vi "Main.vi"() -> ()   [LabVIEW 2020]
uses:
  Serial Settings.ctl
  Data Cluster.ctl
  Main Events.ctl
  <vilib>/Utility/NIReport.llb/Report Type.ctl
  bd07f4a1-b671-4ede-a250-6e16bfbd43fa.vi
  <vilib>/Instr/_visa.llb/VISA Configure Serial Port (Instr).vi
  <vilib>/Utility/file.llb/Write Delimited Spreadsheet (string).vi
  <vilib>/addons/_office/excel.llb/Excel Get Data ([str]).vi
  <vilib>/Comparison/Equal/Equal Functor/Equal Functor.lvclass
  <vilib>/Utility/NIReport.llb/NI_report.lvclass
  <vilib>/Utility/NIReport.llb/NI_ReportGenerationCore.lvlib
  <vilib>/addons/_office/NI_ReportGenerationToolkit.lvlib
  <vilib>/Utility/NIReport.llb/Excel/NI_Excel.lvclass
panel:
  in  "Add Button":bool caption="Start Button"
  in  "Command Data":string
  in  "Select Command":string(combo)
  in  "Create Chain":bool
  in  "Import Script":path
  in  "Save Script Button":bool caption="Start Button"
  out "Imported Commands":string[][](array[string])
  out "CMD Array":T1[](array[typedef])
  out "Data file path":path
  out "Data":string[][](table)=[["Loop", "Step", "Command", "Opcode Sent", "Data Received", "Data Decoded", "Retries", "Time (ms)", "Error"]]
  in  "Timeout (ms)":dbl=1000.0
  out "Script":string[][](table)
  in  "Serial Settings":T2={"baud rate"=115200, "data bits"=8, "parity"=enum."None", "stop bits"=10, "flow control"=0} {"flow control" items=["None"=0, "XON/XOFF"=1, "RTS/CTS"=2, "DTR/DSR"=4]; "stop bits" items=["1.0"=10, "1.5"=15, "2.0"=20]; "data bits" min=5 max=8 step=1; "baud rate" items=["75"=75, "110"=110, "134"=134, "150"=150, "300"=300, "600"=600, "1200"=1200, "1800"=1800, "2400"=2400, "4800"=4800, "7200"=7200, "9600"=9600, "14400"=14400, "19200"=19200, "28800"=28800, "38400"=38400, "56000"=56000, "57600"=57600, "115200"=115200, "128000"=128000, "230400"=230400]}
  in  "Stop Button":bool caption="Start Button"
  in  "Clear Button":bool caption="Start Button"
  out "Status":string
  in  "Start Button":bool
  in  "Number of Retries":u16=3
  in  "Number of Loops":u16=1
  out "COM Port LED":bool
  in  "Select COM Port":refnum<visa-resource-name>
  out "error out":errorcluster
  in  "error in":errorcluster
  # "Create Scipt"
  # "Send Data:"
  # "Receive Data:"
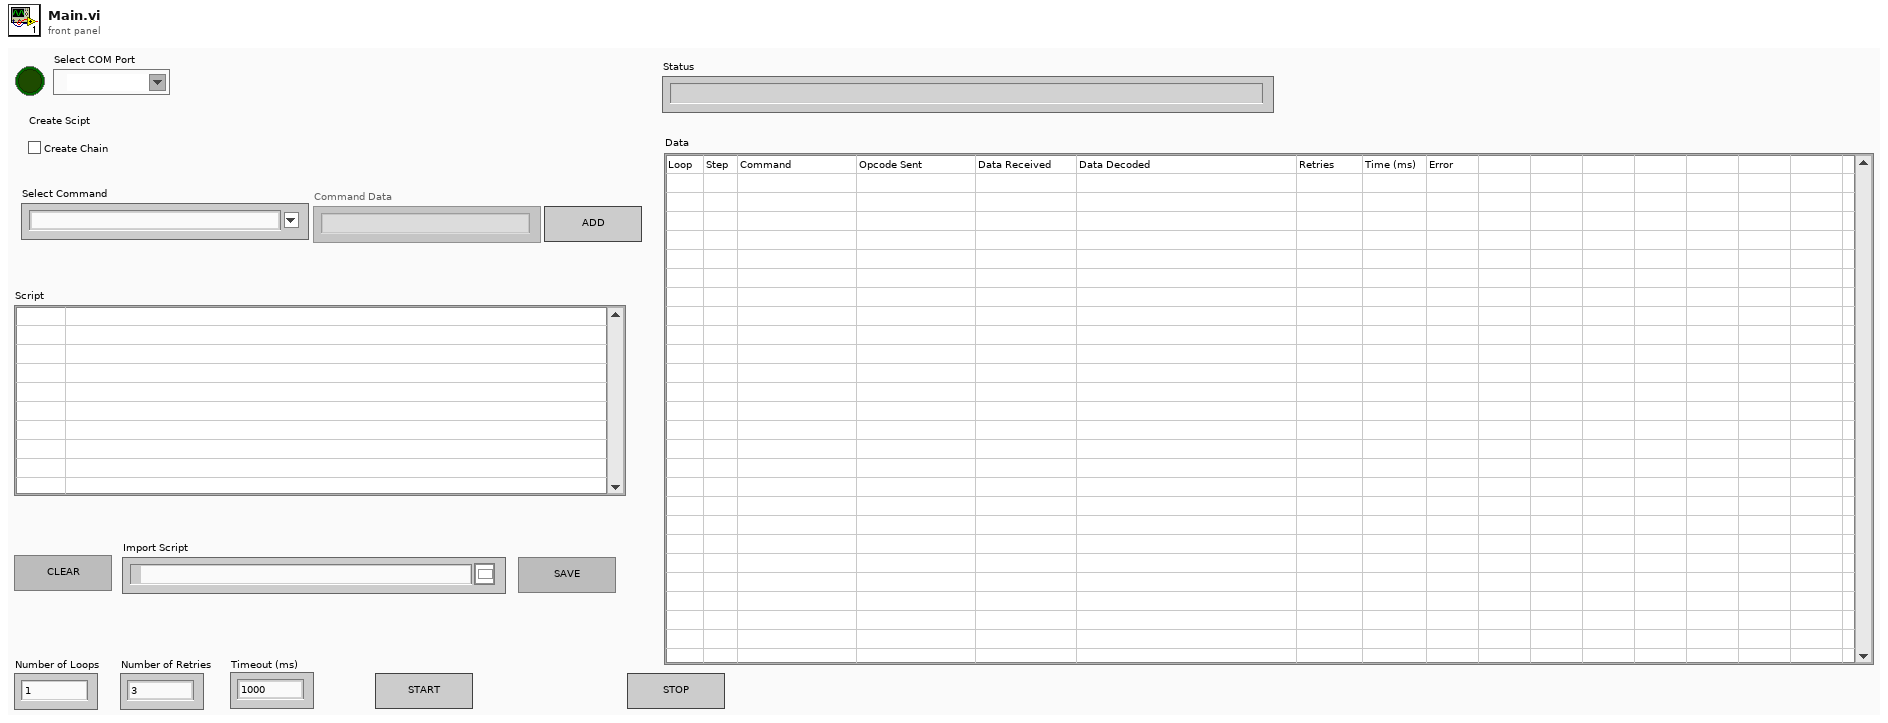
[diagram p1: front panel]
types:
  T1 = typedef "Data Cluster.ctl" = cluster{"Command Name":string, "Command Opcode ":string, "Step":dbl, "Loop":dbl, "Expected Response Size (bytes)":u16, "Number of cmds":dbl, "Data Received (byte array)":u8[], "Retries Executed":u16, "Time (ms)":u16, "Pass?":bool, "Opcode (off) / Instruction (on)":bool, "Data Received String (decoded)":string, "Error":string}
  T2 = typedef "Serial Settings.ctl" = cluster{"baud rate":u32, "data bits":u16, "parity":enum16{"None", "Odd", "Even", "Mark", "Space"}, "stop bits":u16, "flow control":u16}
  T3 = typedef "Main Events.ctl" = enum16{"Default", "Initialize cmds", "Initialize Data File", "Initialize COM Port", "Run Commands", "Save Data File", "End"}
  T4 = typedef "NI_ReportGenerationCore.lvlib/Report Type.ctl" = enum16{"HTML", "Word", "Excel"}
  T5 = enum8{"Enabled", "Disabled", "Disabled and Grayed Out"}
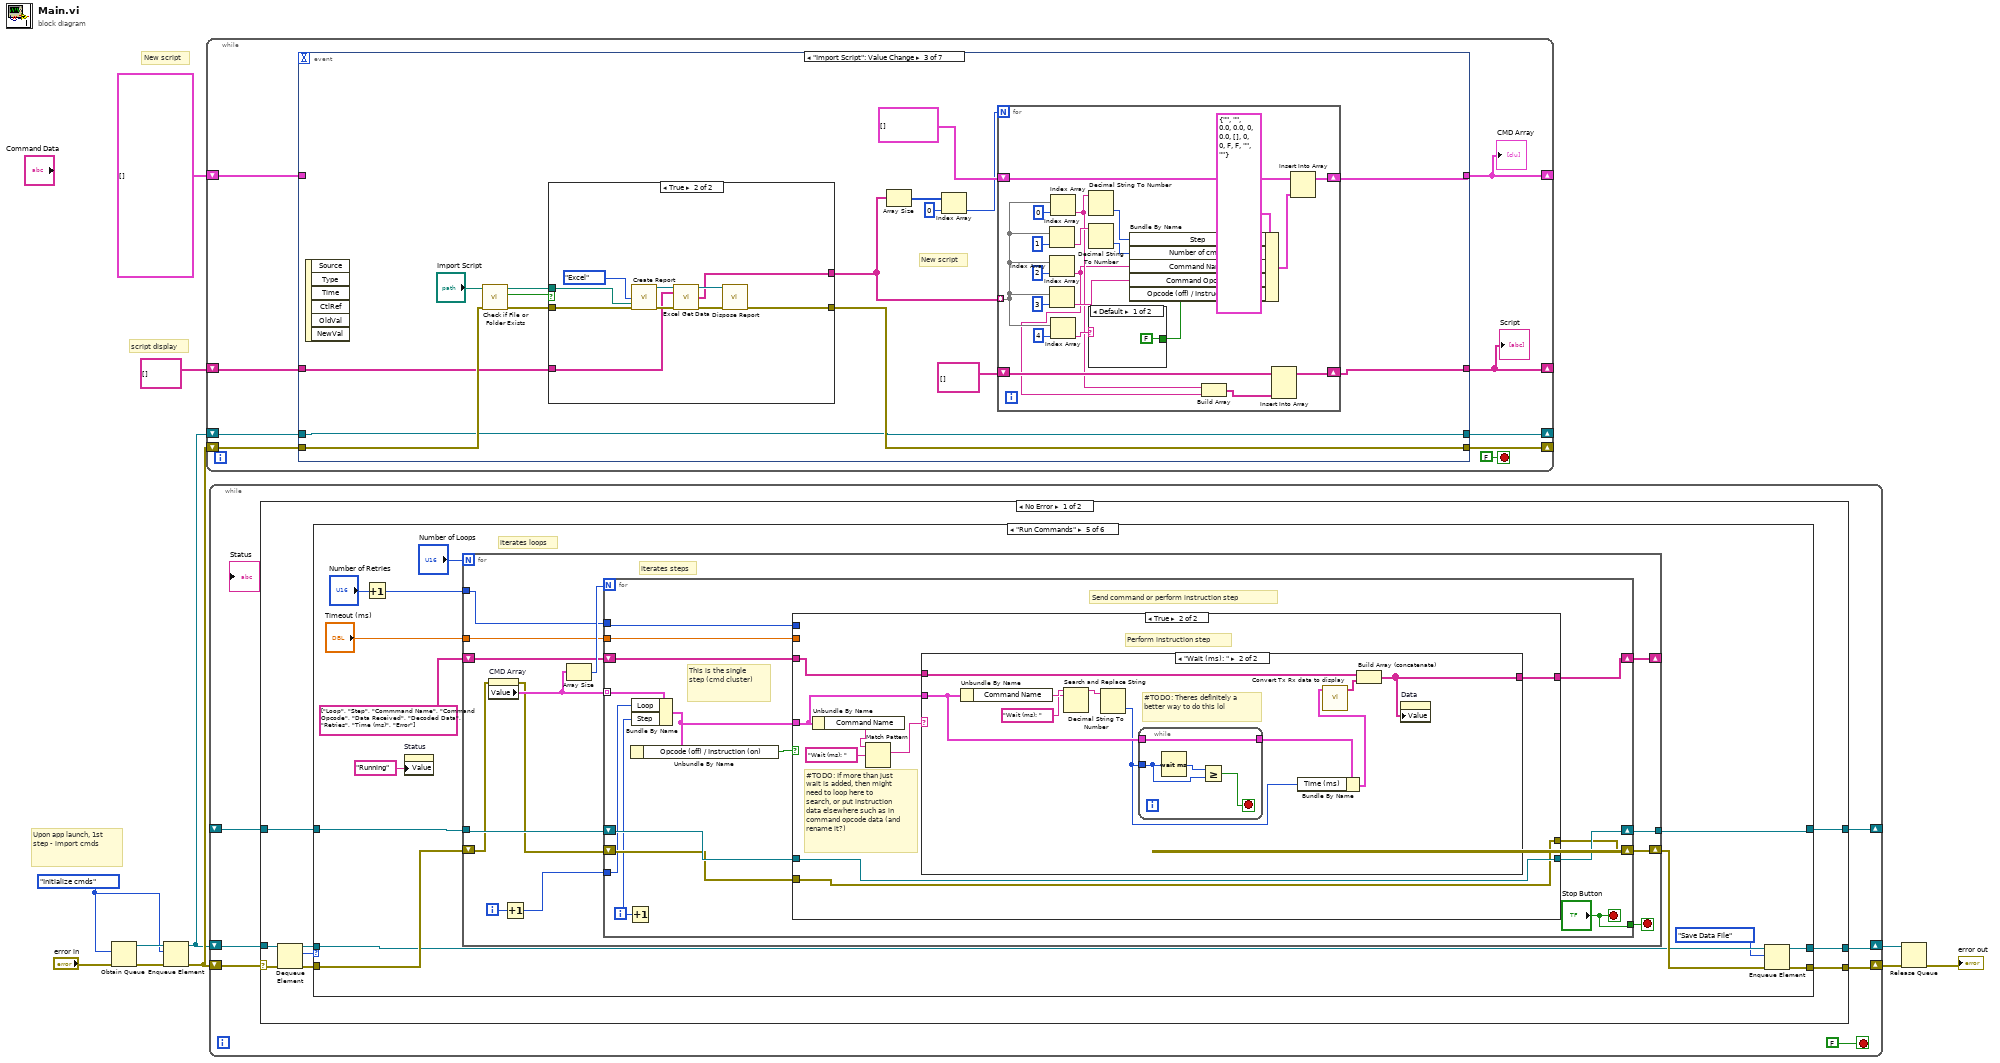
[diagram p0: block diagram]
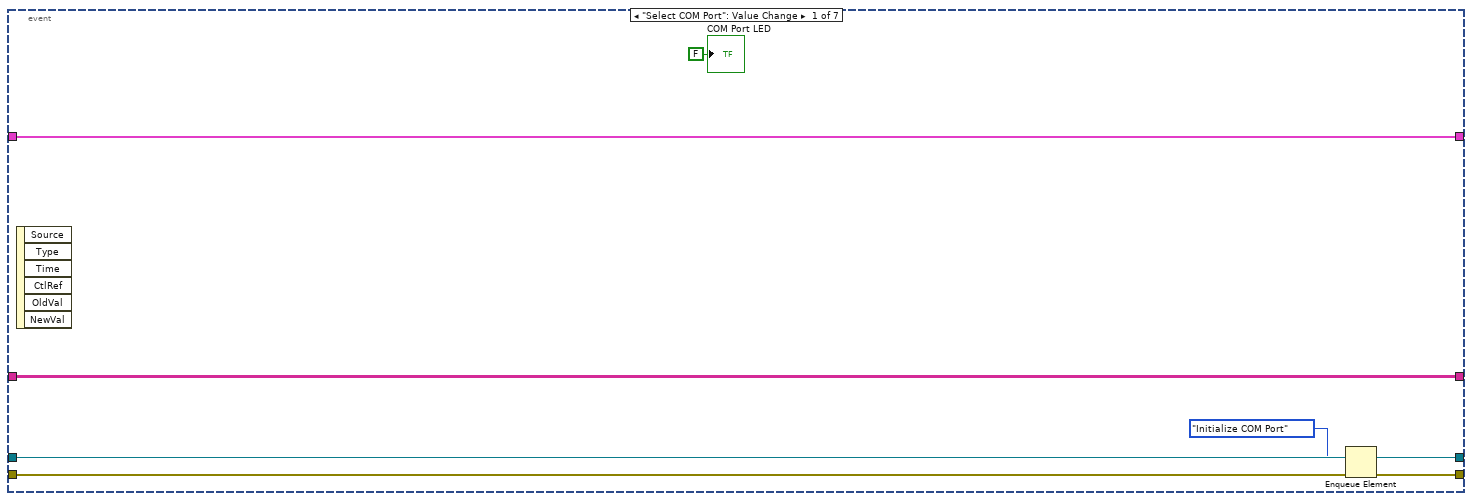
[diagram p2: hidden frame]
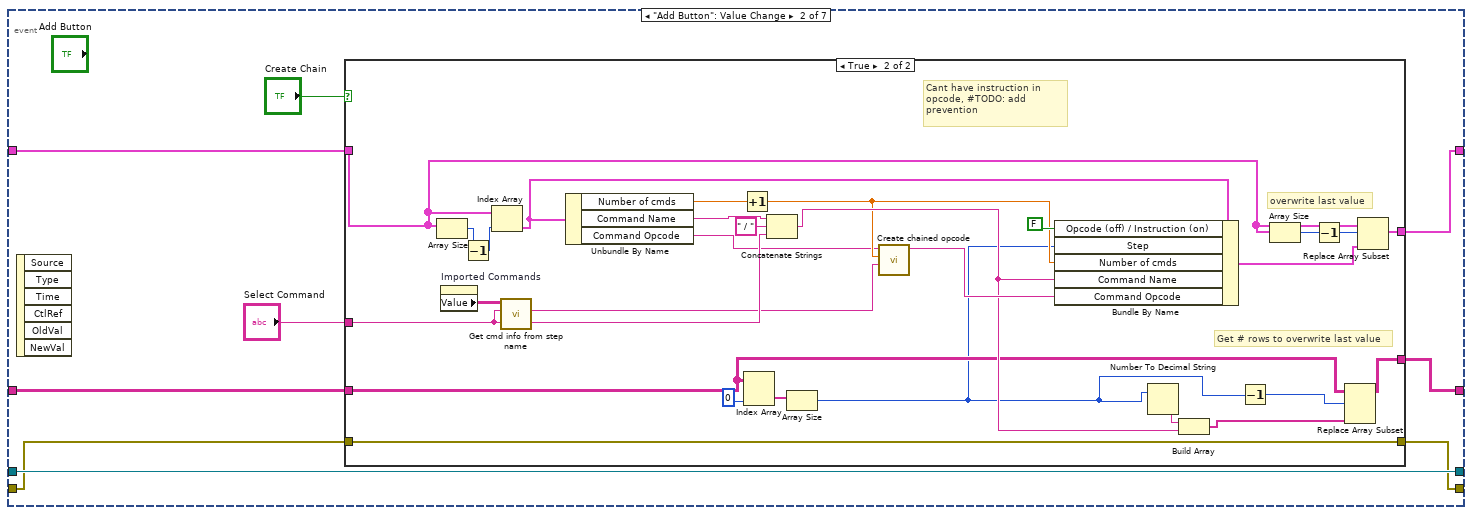
[diagram p3: hidden frame]
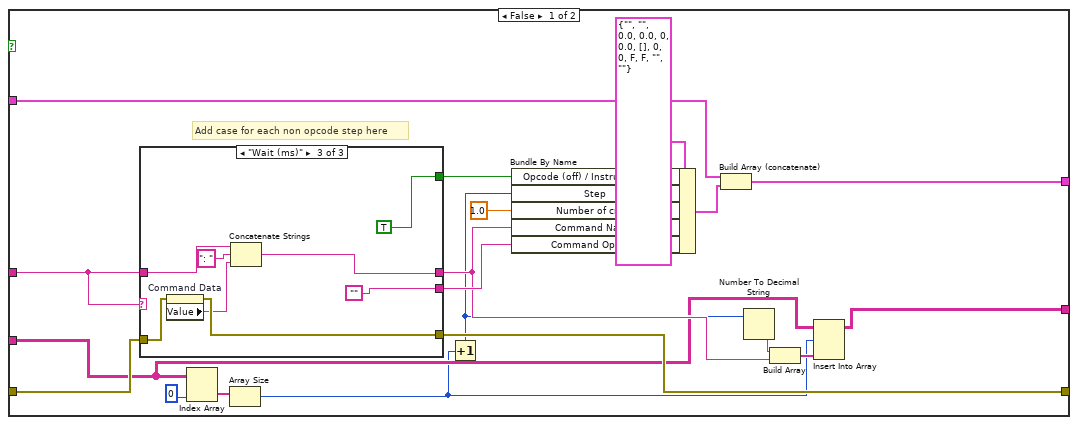
[diagram p4: hidden frame]
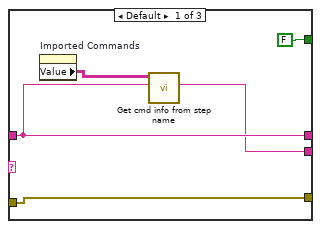
[diagram p5: hidden frame]
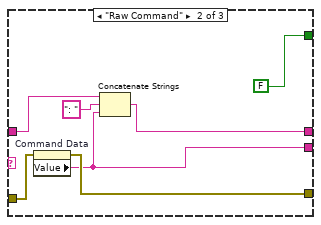
[diagram p6: hidden frame]
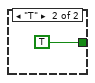
[diagram p7: hidden frame]
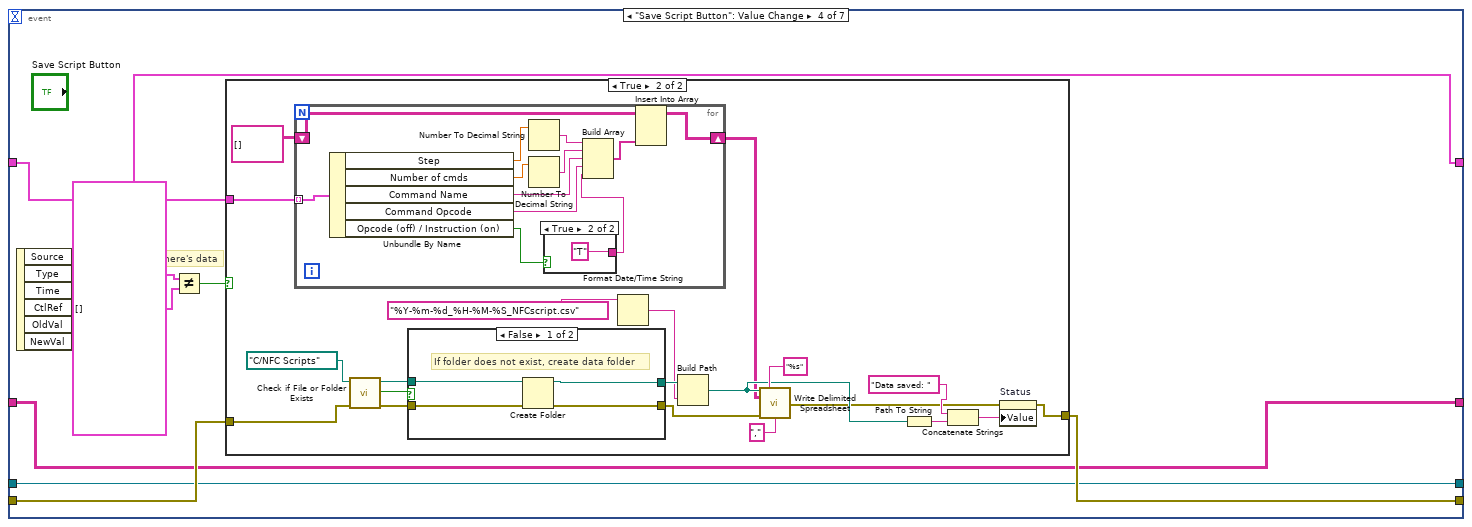
[diagram p9: hidden frame]
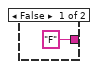
[diagram p11: hidden frame]
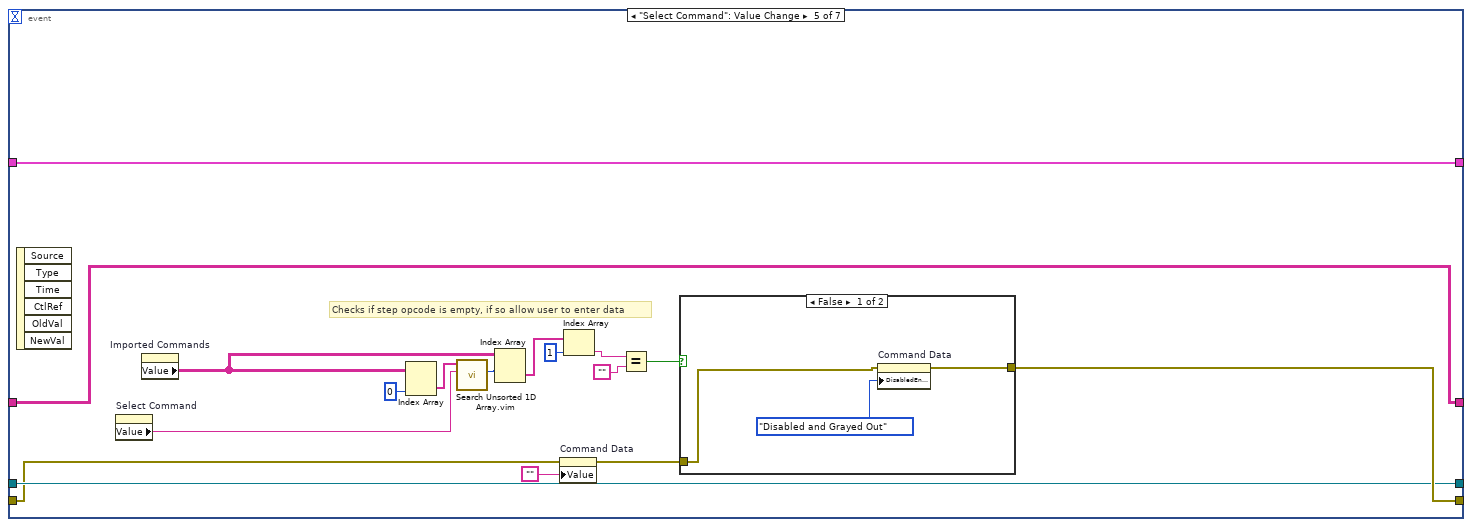
[diagram p13: hidden frame]
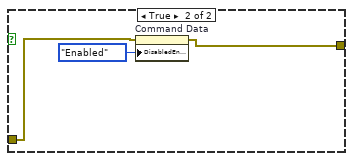
[diagram p14: hidden frame]
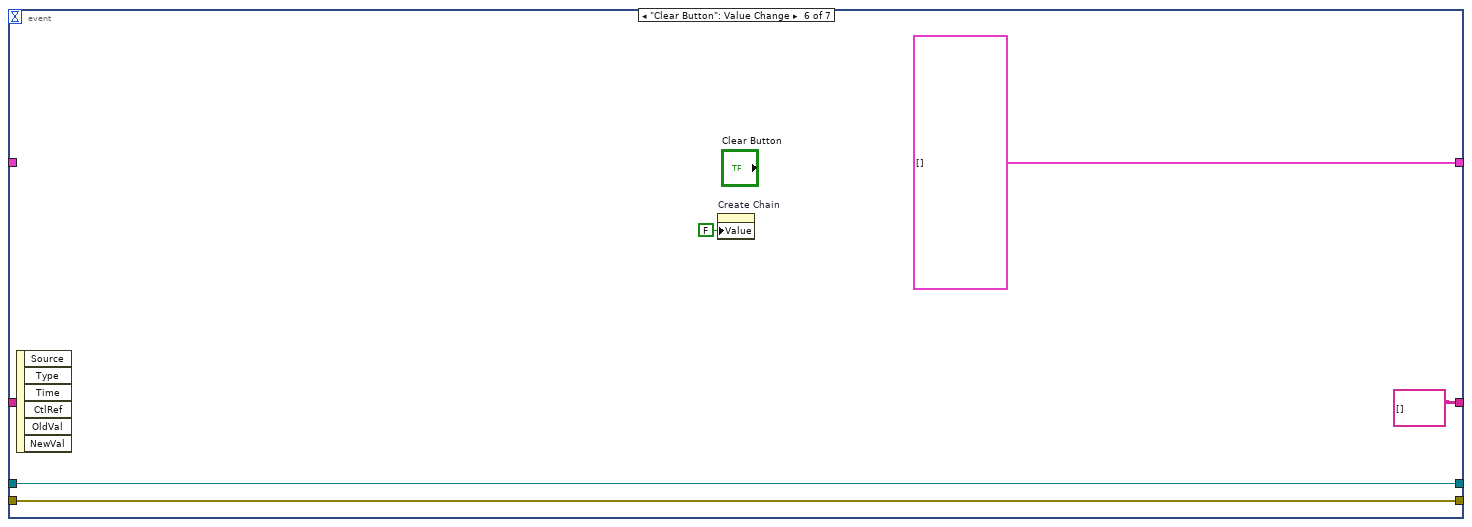
[diagram p15: hidden frame]
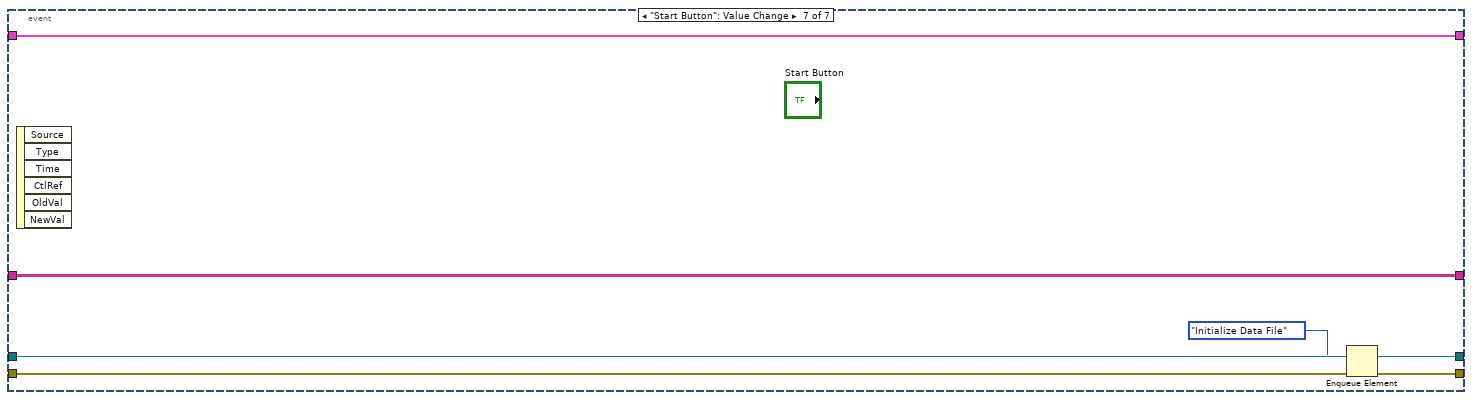
[diagram p16: hidden frame]
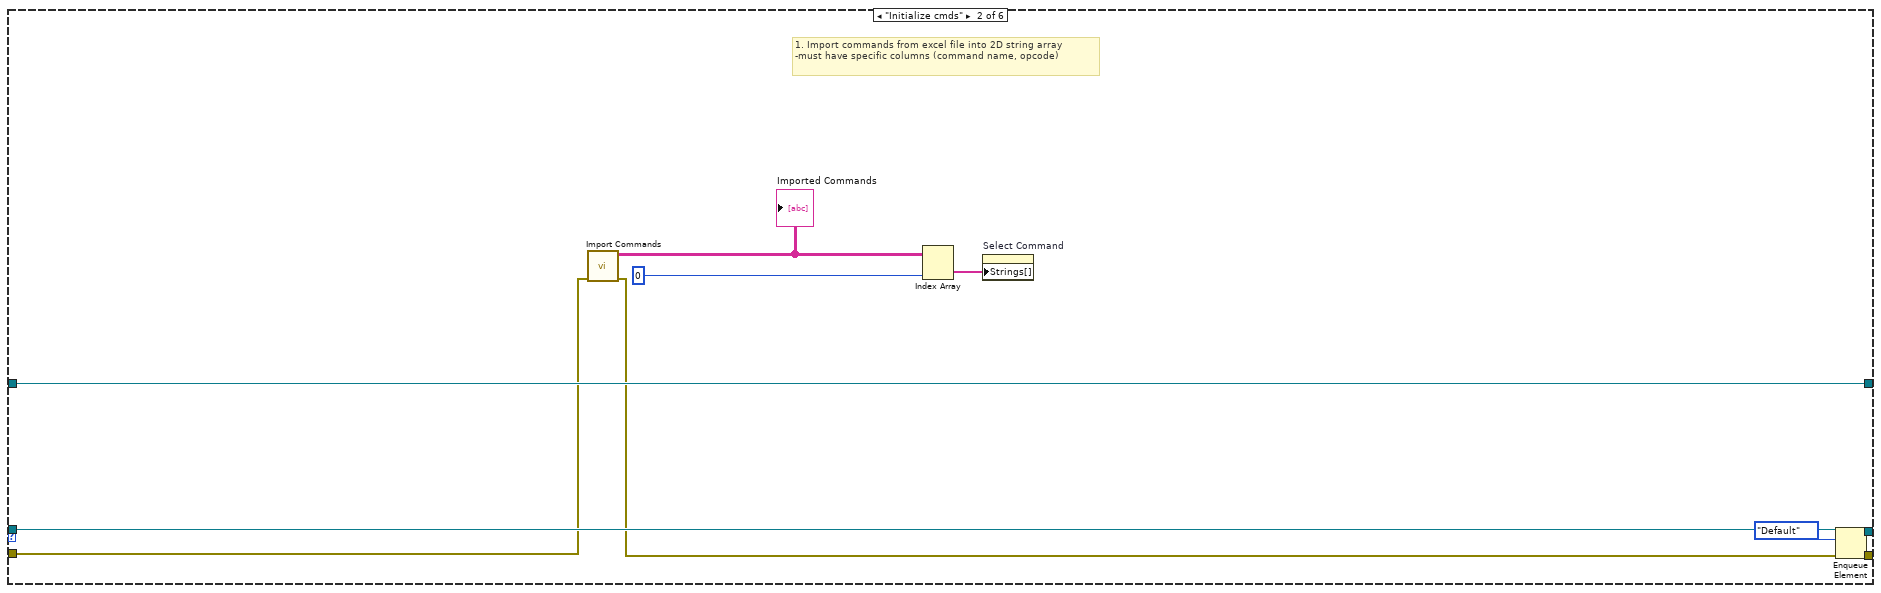
[diagram p18: hidden frame]
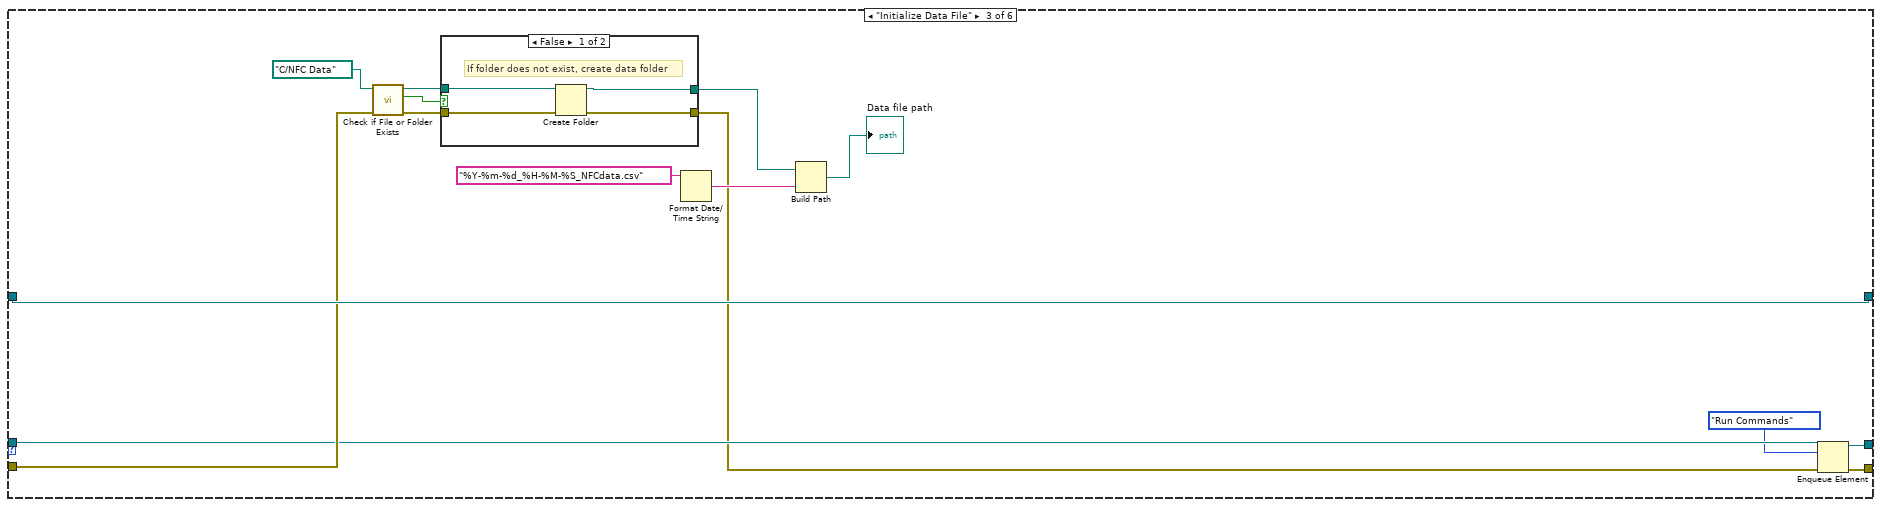
[diagram p19: hidden frame]
diagram:
  w3 = Main_Events."Initialize cmds" ("Main Enum")
  # "script display"
  # "New script"
  # "Upon app launch, 1st step - import cmds"
  n1 = Obtain Queue(element data type=w3, error in (no error)="error in") -> (queue out=w7:refnum<queue>, error out=w10:errorcluster)  [unwired: 3 in, 1 out]
  n2 = Enqueue Element(queue=w7, element=w3, error in (no error)=w10) -> (queue out=w4:refnum<queue>, error out=w5:errorcluster)  [unwired: 1 in, 1 out]
  n3 = while {
    shift-right: [w19] -> _
    shift-left: w5 -> [w20]
    shift-right: [w17] -> _
    shift-left: w4 -> [w18]
    shift-right: [w12] -> _
    shift-left: T1[] [] ("Array") -> [w15]
    shift-right: [w13] -> _
    shift-left: string[][] [] ("Script") -> [w14]
    stop <- FALSE stop-if-true
    n4 = event shown="[2] \"Import Script\": Value Change" {
      selector: _ -> [_ _ _ _ _ _ _]
      dyn-events: _ -> [_ _ _ _ _ _ _]
      timeout: _ -> [_ _ _ _ _ _ _]
      tunnel: w20 -> [w24 w34 w116 w161 w205 w229 w236]
      tunnel: [w28 w33 w114 w160 w220 w229 w237] -> w19
      tunnel: w18 -> [w27 w35 w113 w159 w219 w230 w235]
      tunnel: [w26 w35 w113 w159 w219 w230 w238] -> w17
      tunnel: w15 -> [w22 w32 _ w156 w218 _ w233]
      tunnel: [w22 w31 w110 w156 w218 T1[] [] ("Array") w233] -> w12
      tunnel: w14 -> [w21 w30 w115 w158 w217 _ w232]
      tunnel: [w21 w29 w108 w158 w217 string[][] [] ("Script") w232] -> w13
      event "Select COM Port": Value Change {
        n5 = event-data() -> ()  [unwired: 1 in, 6 out]
        n6 = Enqueue Element(queue=w27, element=Main_Events."Initialize COM Port" ("Main Enum"), error in (no error)=w24) -> (queue out=w26:refnum<queue>, error out=w28:errorcluster)  [unwired: 1 in, 1 out]
        "COM Port LED" <- FALSE ("COM Port LED")
      }
      event "Add Button": Value Change {
        n7 = event-data() -> ()  [unwired: 1 in, 6 out]
        n8 = case shown="True" "Create Chain" {
          tunnel: "Select Command" -> [w56 w83]
          tunnel: w34 -> [w55 w103]
          tunnel: [w54 w103] -> w33
          tunnel: w32 -> [w48 w99]
          tunnel: [w47 w97] -> w31
          tunnel: w30 -> [w40 w88]
          tunnel: [w39 w89] -> w29
          frame False {
            # "Add case for each non opcode step here"
            n9 = case shown="\"Wait (ms)\"" w56 {
              tunnel: [w58 w66 w74] -> w44
              tunnel: w56 -> [w58 w68 w76]
              tunnel: [w57 w63 ""] -> w51
              tunnel: w55 -> [w61 w65 w73]
              tunnel: [w61 w64 w72] -> w54
              tunnel: [FALSE ("Opcode (off) / Instruction (on)") FALSE ("Opcode (off) / Instruction (on)") TRUE ("Opcode (off) / Instruction (on)")] -> w50
              frame Default {
                n10 = property on="Imported Commands" class="Arr (strict)"() -> ("Value"=w59:string[][])  [unwired: 2 in, 2 out]
                n11 = call "Get cmd info from step name.vi"("Select Command"=w58, "Command Library Data"=w59) -> ("cmd opcode (string)"=w57:string)  [unwired: 8 in, 1 out]
              }
              frame "Raw Command" {
                n12 = property on="Command Data" class="Str"(error in=w65) -> (error out=w64:errorcluster, "Value"=w63:string)  [unwired: 1 in, 1 out]
                n13 = Concatenate Strings(w68, ": " ("string"), w63) -> (w66:string)
              }
              frame "Wait (ms)" {
                n14 = property on="Command Data" class="Str"(error in=w73) -> (error out=w72:errorcluster, "Value"=w71:string)  [unwired: 1 in, 1 out]
                n15 = Concatenate Strings(w76, ": " ("string"), w71) -> (w74:string)
              }
            }
            n16 = Index Array(array=w40, index (col)=0 ("index")) -> (element=w42:string[])  [unwired: 1 in]
            n17 = Array Size(array=w42) -> (size(s)=w38:i32)
            n18 = Increment(x=w38) -> (x+1=w41:i32)
            n19 = Bundle By Name(cluster=T1 {"Command Name"="", "Command Opcode "="", "Step"=0.0, "Loop"=0.0, "Expected Response Size (bytes)"=0, "Number of cmds"=0.0, "Data Received (byte array)"=[], "Retries Executed"=0, "Time (ms)"=0, "Pass?"=FALSE, "Opcode (off) / Instruction (on)"=FALSE, "Data Received String (decoded)"="", "Error"=""} ("Data Cluster"), "Opcode (off) / Instruction (on)"=w50, "Step"=w41, "Number of cmds"=1.0, "Command Name"=w44, "Command Opcode"=w51) -> (w53:T1)
            n20 = Build Array (concatenate)(w48, w53) -> (w47:T1[])
            n21 = Number To Decimal String(number=w41) -> (decimal integer string=w46:string)  [unwired: 1 in]
            n22 = Build Array(w46, w44) -> (w45:string[])
            n23 = Insert Into Array(array=w40, index (row)=w38, new element=w45) -> (w39:string[][])  [unwired: 1 in]
          }
          frame True {
            # "Cant have instruction in opcode, #TODO: add prevention"
            # "Get # rows to overwrite last value"
            # "overwrite last value"
            n24 = Array Size(array=w99) -> (size(s)=w93:i32)
            n25 = property on="Imported Commands" class="Arr (strict)"() -> ("Value"=w84:string[][])  [unwired: 2 in, 2 out]
            n26 = Decrement(x=w93) -> (x-1=w92:i32)
            n27 = Index Array(array=w99, index=w92) -> (element=w96:T1)
            n28 = call "Get cmd info from step name.vi"("Select Command"=w83, "Command Library Data"=w84) -> ("cmd opcode (string)"=w81:string)  [unwired: 8 in, 1 out]
            n29 = Unbundle By Name(w96) -> ("Number of cmds"=w82:dbl, "Command Name"=w102:string, "Command Opcode"=w79:string)
            n30 = Increment(x=w82) -> (x+1=w80:dbl)
            n31 = Index Array(array=w88, index (col)=0 ("index")) -> (element=w86:string[])  [unwired: 1 in]
            n32 = Concatenate Strings(w102, " / " ("string"), w83) -> (w90:string)
            n33 = Array Size(array=w86) -> (size(s)=w78:i32)
            n34 = call "Create chained opcode.vi"("new cmd opcode"=w81, "Number of commands"=w80, "Current cmd opcode"=w79) -> ("new chained opcode"=w100:string)  [unwired: 8 in]
            n35 = Bundle By Name(cluster=w96, "Opcode (off) / Instruction (on)"=FALSE, "Step"=w78, "Number of cmds"=w80, "Command Name"=w90, "Command Opcode"=w100) -> (w98:T1)
            n36 = Number To Decimal String(number=w78) -> (decimal integer string=w91:string)  [unwired: 1 in]
            n37 = Build Array(w91, w90) -> (w85:string[])
            n38 = Decrement(x=w78) -> (x-1=w77:i32)
            n39 = Array Size(array=w99) -> (size(s)=w95:i32)
            n40 = Decrement(x=w95) -> (x-1=w94:i32)
            n41 = Replace Array Subset(array=w88, new element=w85, index (row)=w77) -> (w89:string[][])  [unwired: 1 in]
            n42 = Replace Array Subset(array=w99, new element=w98, index=w94) -> (w97:T1[])
          }
        }
      }
      event "Import Script": Value Change {
        # "New script"
        n43 = event-data() -> ()  [unwired: 1 in, 6 out]
        n44 = call <vilib>:"Check if File or Folder Exists.vi"("error in (no error)"=w116, "path"="Import Script") -> ("error out"=w117:errorcluster, "file or folder exists?"=w119:bool, "dup path"=w118:path)  [unwired: 7 in]
        n45 = case shown="True" w119 {
          tunnel: [w144 w146] -> w107
          tunnel: [w145 w154] -> w114
          tunnel: w118 -> [_ w149]
          tunnel: w117 -> [w145 w148]
          tunnel: w115 -> [w144 w147]
          frame False {
          }
          frame True {
            n46 = call <vilib>:"Create Report.vi"("report type"=Report_Type."Excel", "template (empty)"=w149, "error in (no error)"=w148) -> ("report out"=w153:refnum<class "NI_report.lvclass">, "error out"=w151:errorcluster)  [unwired: 11 in]
            n47 = call-poly <vilib>:"Excel Get Data.vi"("report in"=w153, "data type"=w147, "error in (no error)"=w151) -> ("report out"=w152:refnum<class "NI_report.lvclass">, "data"=w146:string[][], "error out"=w150:errorcluster)  [unwired: 10 in]
            n48 = call-dynamic "Dispose Report.vi"("report in"=w152, "error in (no error)"=w150) -> ("error out"=w154:errorcluster)  [unwired: 13 in]
          }
        }
        n49 = Array Size(array=w107) -> (size(s)=w106:i32[])
        n50 = Index Array(array=w106, index=0) -> (element=w105:i32)
        n51 = for {
          N: w105 -> [_]
          tunnel: w107 -> [w136] mode=indexing
          shift-right: [w126] -> w110
          shift-left: T1[] [] ("Array") -> [w128]
          shift-right: [w125] -> w108
          shift-left: string[][] [] ("Script") -> [w124]
          n52 = Index Array(array=w136, index=1) -> (element=w133:string)
          n53 = Index Array(array=w136, index=2) -> (element=w122:string)
          n54 = Index Array(array=w136, index=3) -> (element=w134:string)
          n55 = Index Array(array=w136, index=0) -> (element=w123:string)
          n56 = Index Array(array=w136, index=4) -> (element=w130:string)
          n57 = Decimal String To Number(string=w123) -> (number=w131:i32)  [unwired: 2 in, 1 out]
          n58 = Decimal String To Number(string=w133) -> (number=w132:i32)  [unwired: 2 in, 1 out]
          n59 = case shown="Default" w130 {
            tunnel: [FALSE TRUE] -> w129
            frame Default {
            }
            frame "T" {
            }
          }
          n60 = Bundle By Name(cluster=T1 {"Command Name"="", "Command Opcode "="", "Step"=0.0, "Loop"=0.0, "Expected Response Size (bytes)"=0, "Number of cmds"=0.0, "Data Received (byte array)"=[], "Retries Executed"=0, "Time (ms)"=0, "Pass?"=FALSE, "Opcode (off) / Instruction (on)"=FALSE, "Data Received String (decoded)"="", "Error"=""} ("Data Cluster"), "Step"=w131, "Number of cmds"=w132, "Command Name"=w122, "Command Opcode"=w134, "Opcode (off) / Instruction (on)"=w129) -> (w127:T1)
          n61 = Build Array(w123, w122) -> (w121:string[])
          n62 = Insert Into Array(array=w124, new element=w121) -> (w125:string[][])  [unwired: 2 in]
          n63 = Insert Into Array(array=w128, new element=w127) -> (w126:T1[])  [unwired: 1 in]
        }
      }
      event "Save Script Button": Value Change {
        # "If there's data"
        n64 = event-data() -> ()  [unwired: 1 in, 6 out]
        n65 = Not Equal?(x=w156, y=T1[] [] ("Array")) -> (x != y?=w162:bool)
        n66 = case shown="True" w162 {
          tunnel: w161 -> [w163 w176]
          tunnel: [w163 w167] -> w160
          tunnel: w156 -> [_ w166]
          frame False {
          }
          frame True {
            n67 = for {
              tunnel: w166 -> [w195] mode=indexing
              shift-right: [w192] -> w164
              shift-left: string[][] [] ("Script") -> [w193]
              n68 = Unbundle By Name(w195) -> ("Step"=w191:dbl, "Number of cmds"=w190:dbl, "Command Name"=w187:string, "Command Opcode"=w186:string, "Opcode (off) / Instruction (on)"=w185:bool)
              n69 = Number To Decimal String(number=w191) -> (decimal integer string=w189:string)  [unwired: 1 in]
              n70 = Number To Decimal String(number=w190) -> (decimal integer string=w188:string)  [unwired: 1 in]
              n71 = case shown="True" w185 {
                tunnel: ["F" "T"] -> w184
                frame False {
                }
                frame True {
                }
              }
              n72 = Build Array(w189, w188, w187, w186, w184) -> (w194:string[])
              n73 = Insert Into Array(array=w193, new element=w194) -> (w192:string[][])  [unwired: 2 in]
            }
            n74 = call <vilib>:"Check if File or Folder Exists.vi"("error in (no error)"=w176, "path"=path "C:/NFC Scripts") -> ("error out"=w181:errorcluster, "file or folder exists?"=w183:bool, "dup path"=w182:path)  [unwired: 7 in]
            n75 = case shown="False" w183 {
              tunnel: w182 -> [w201 w203]
              tunnel: w181 -> [w200 w202]
              tunnel: [w199 w203] -> w179
              tunnel: [w198 w202] -> w171
              frame False {
                # "If folder does not exist, create data folder"
                n76 = Create Folder(path (use dialog)=w201, error in=w200) -> (created path=w199:path, error out=w198:errorcluster)  [unwired: 1 in, 1 out]
              }
              frame True {
              }
            }
            n77 = Format Date/Time String(time format string (%c)="%Y-%m-%d_%H-%M-%S_NFCscript.csv") -> (date/time string=w178:string)  [unwired: 2 in]
            n78 = Build Path(base path=w179, name or relative path=w178) -> (appended path=w170:path)
            n79 = call-poly <vilib>:"Write Delimited Spreadsheet.vi"("file path (dialog if empty)"=w170, "format (%s)"="%s", "2D data"=w164, "error in (no error)"=w171, "delimiter (\\t)"="," ("delimiter (\\t)")) -> ("error out"=w169:errorcluster)  [unwired: 9 in, 1 out]
            n80 = Path To String(path=w170) -> (string=w173:string)
            n81 = Concatenate Strings("Data saved: " ("Status"), w173) -> (w168:string)
            n82 = property on="Status" class="Str"(error in=w169, "Value"=w168) -> (error out=w167:errorcluster)  [unwired: 1 in, 1 out]
          }
        }
      }
      event "Select Command": Value Change {
        # "Checks if step opcode is empty, if so allow user to enter data"
        n83 = event-data() -> ()  [unwired: 1 in, 6 out]
        n84 = property on="Select Command" class="CmbBox"() -> ("Value"=w210:string)  [unwired: 2 in, 2 out]
        n85 = property on="Imported Commands" class="Arr (strict)"() -> ("Value"=w211:string[][])  [unwired: 2 in, 2 out]
        n86 = Index Array(array=w211, index (col)=0 ("disabled index (col)")) -> (element=w215:string[])  [unwired: 1 in]
        n87 = call "Search Unsorted 1D Array.vim"("element"=w210, "unsorted 1D array"=w215) -> ("index of element"=w216:i32)  [unwired: 9 in]
        n88 = Index Array(array=w211, index (row)=w216) -> (element=w212:string[])  [unwired: 1 in]
        n89 = property on="Command Data" class="Str"(error in=w205, "Value"="") -> (error out=w204:errorcluster)  [unwired: 1 in, 1 out]
        n90 = Index Array(array=w212, index=1) -> (element=w209:string)
        n91 = Equal?(x=w209, y="") -> (x = y?=w207:bool)
        n92 = case shown="False" w207 {
          tunnel: w204 -> [w221 w225]
          tunnel: [w222 w224] -> w220
          frame False {
            n93 = property on="Command Data" class="Str"(error in=w221, "DisabledEnum"=T5."Disabled and Grayed Out" ("Disabled")) -> (error out=w222:errorcluster)  [unwired: 1 in, 1 out]
          }
          frame True {
            n94 = property on="Command Data" class="Str"(error in=w225, "DisabledEnum"=T5."Enabled" ("Disabled")) -> (error out=w224:errorcluster)  [unwired: 1 in, 1 out]
          }
        }
      }
      event "Clear Button": Value Change {
        n95 = event-data() -> ()  [unwired: 1 in, 6 out]
        n96 = property on="Create Chain" class="Bool (strict)"("Value"=FALSE ("Create Chain")) -> ()  [unwired: 2 in, 2 out]
      }
      event "Start Button": Value Change {
        n97 = event-data() -> ()  [unwired: 1 in, 6 out]
        n98 = Enqueue Element(queue=w235, element=Main_Events."Initialize Data File", error in (no error)=w236) -> (queue out=w238:refnum<queue>, error out=w237:errorcluster)  [unwired: 1 in, 1 out]
      }
    }
    "Script" <- w13
    "CMD Array" <- w12
  }
  n99 = while {
    shift-right: [w243] -> w9
    shift-left: w5 -> [w245]
    shift-right: [w242] -> w6
    shift-left: w4 -> [w244]
    shift-right: [w241] -> _
    shift-left: _ -> [w240]
    stop <- FALSE stop-if-true
    n100 = case shown="No Error" w245 {
      selector: w245 -> [w253 w427]
      tunnel: w244 -> [w252 w428]
      tunnel: [w249 w427] -> w243
      tunnel: [w248 w428] -> w242
      tunnel: [w247 w426] -> w241
      tunnel: w240 -> [w246 w426]
      frame No Error {
        n101 = Dequeue Element(queue=w252, error in (no error)=w253) -> (queue out=w250:refnum<queue>, element=w251:T3, error out=w254:errorcluster)  [unwired: 1 in, 1 out]
        n102 = case shown="\"Run Commands\"" w251 {
          tunnel: w254 -> [w256 w262 w279 w300 w329 w422]
          tunnel: w250 -> [w257 w266 w272 w299 w324 w423]
          tunnel: [w256 w267 w273 w289 w326 w414] -> w249
          tunnel: [w257 w265 w274 w292 w327 w423] -> w248
          tunnel: [w255 w263 w282 w291 w330 w424] -> w247
          tunnel: w246 -> [w255 w263 w282 _ w331 w424]
          frame "Default", Default {
          }
          frame "Initialize cmds" {
            # "1. Import commands from excel file into 2D string array\n-must have specific columns (command name, opcode)"
            n103 = call "Import Commands.vi"("error in"=w262) -> ("error out"=w261:errorcluster, "Imported Commands"=w258:string[][])  [unwired: 9 in]
            "Imported Commands" <- w258
            n104 = Index Array(array=w258, index (col)=0 ("disabled index (col)")) -> (element=w259:string[])  [unwired: 1 in]
            n105 = property on="Select Command" class="CmbBox"("Strings[]"=w259) -> ()  [unwired: 2 in, 2 out]
            n106 = Enqueue Element(queue=w266, element=Main_Events."Default" ("Main Enum"), error in (no error)=w261) -> (queue out=w265:refnum<queue>, error out=w267:errorcluster)  [unwired: 1 in, 1 out]
          }
          frame "Initialize Data File" {
            n107 = call <vilib>:"Check if File or Folder Exists.vi"("error in (no error)"=w279, "path"=path "C:/NFC Data") -> ("error out"=w278:errorcluster, "file or folder exists?"=w281:bool, "dup path"=w280:path)  [unwired: 7 in]
            n108 = case shown="False" w281 {
              tunnel: w280 -> [w286 w288]
              tunnel: w278 -> [w285 w287]
              tunnel: [w284 w288] -> w276
              tunnel: [w283 w287] -> w268
              frame False {
                # "If folder does not exist, create data folder"
                n109 = Create Folder(path (use dialog)=w286, error in=w285) -> (created path=w284:path, error out=w283:errorcluster)  [unwired: 1 in, 1 out]
              }
              frame True {
              }
            }
            n110 = Format Date/Time String(time format string (%c)="%Y-%m-%d_%H-%M-%S_NFCdata.csv") -> (date/time string=w275:string)  [unwired: 2 in]
            n111 = Build Path(base path=w276, name or relative path=w275) -> (appended path=→"Data file path":path)
            n112 = Enqueue Element(queue=w272, element=Main_Events."Run Commands", error in (no error)=w268) -> (queue out=w274:refnum<queue>, error out=w273:errorcluster)  [unwired: 1 in, 1 out]
          }
          frame "Initialize COM Port" {
            # "If there's any error at this point, it's displayed and cleared. This assumes the error is com related and then clears all errors"
            # "Configure the serial port and wait 1 sec."
            n113 = Unbundle By Name("Serial Settings") -> ("baud rate"=w297:u32, "data bits"=w294:u16, "parity"=w296:enum16{"None", "Odd", "Even", "Mark", "Space"}, "stop bits"=w295:u16)
            n114 = call-poly "VISA Configure Serial Port"("VISA resource name"="Select COM Port", "Enable Termination\nChar (T)"=FALSE ("Enable Termination\nChar (T)"), "baud rate (9600)"=w297, "data bits (8)"=w294, "parity (0:none)"=w296, "error in (no error)"=w300, "stop bits (10: 1 bit)"=w295) -> ("VISA resource name out"=w298:refnum<visa-resource-name>, "error out"=w303:errorcluster)  [unwired: 7 in]
            n115 = call "Time Delay"("error in (no error)"=w303, "Delay Time (s)"=1.0) -> ("error out"=w290:errorcluster)  [unwired: 9 in]
            n116 = case shown="No Error" w290 {
              selector: w290 -> [w306 w311]
              tunnel: w299 -> [w309 w316]
              tunnel: [w305 w317] -> w289
              tunnel: [w309 w316] -> w292
              tunnel: [w308 refnum<visa-resource-name> refnum ("VISA resource name out")] -> w291
              tunnel: w298 -> [w308 w315]
              frame No Error {
                # "No COM Error... Continue"
                n117 = property on="COM Port LED" class="Bool (strict)"(error in=w306, "Value"=TRUE ("COM Port LED")) -> (error out=w305:errorcluster)  [unwired: 1 in, 1 out]
              }
              frame Error {
                n118 = property on="COM Port LED" class="Bool (strict)"(error in=w311, "Value"=FALSE ("COM Port LED")) -> (error out=w310:errorcluster)  [unwired: 1 in, 1 out]
                n119 = VISA Close(VISA resource name=w315, error in (no error)=w310) -> (error out=w314:errorcluster)
                n120 = call <vilib>:"Simple Error Handler.vi"("error in (no error)"=w314) -> ("error out"=w318:errorcluster)  [unwired: 4 in, 4 out]
                n121 = call <vilib>:"Clear Errors.vi"("error in (no error)"=w318) -> ("error out"=w317:errorcluster)  [unwired: 5 in, 1 out]
              }
            }
          }
          frame "Run Commands" {
            # "iterates loops"
            n122 = Increment(x="Number of Retries") -> (x+1=w320:u16)
            n123 = property on="Status" class="Str"("Value"="Running" ("Status")) -> ()  [unwired: 2 in, 2 out]
            n124 = for {
              N: "Number of Loops" -> [_]
              tunnel: [w345] -> w330
              tunnel: w331 -> [w343]
              shift-right: [w344] -> w325
              shift-left: w329 -> [w336]
              shift-right: [w339] -> _
              shift-left: string[][] [["Loop", "Step", "Commmand Name", "Command Opcode", "Data Received", "Decoded Data", "Retries", "Time (ms)", "Error"]] ("element") -> [w340]
              tunnel: w320 -> [w334]
              tunnel: "Timeout (ms)" -> [w333]
              i -> [w342]
              stop <- w338 stop-if-true
              # "iterates steps"
              n125 = property on="CMD Array" class="Arr (strict)"(error in=w336) -> (error out=w335:errorcluster, "Value"=w337:T1[])  [unwired: 1 in, 1 out]
              n126 = Increment(x=w342) -> (x+1=w341:i32)
              n127 = Array Size(array=w337) -> (size(s)=w346:i32)
              n128 = for {
                N: w346 -> [_]
                tunnel: w337 -> [w351] mode=indexing
                shift-right: [w359] -> w345
                shift-left: w343 -> [w361]
                shift-right: [w358] -> w344
                shift-left: w335 -> [w360]
                tunnel: w341 -> [w355]
                shift-right: [w353] -> w339
                shift-left: w340 -> [w354]
                tunnel: ["Stop Button"] -> w338
                tunnel: w334 -> [w348]
                tunnel: w333 -> [w347]
                i -> [w357]
                stop <- "Stop Button" stop-if-true
                # "Send command or perform instruction step"
                # "This is the single step (cmd cluster)"
                n129 = Increment(x=w357) -> (x+1=w356:i32)
                n130 = Bundle By Name(cluster=w351, "Loop"=w355, "Step"=w356) -> (w349:T1)
                n131 = Unbundle By Name(w349) -> ("Opcode (off) / Instruction (on)"=w350:bool)
                n132 = case shown="True" w350 {
                  tunnel: w361 -> [w370 w395]
                  tunnel: w360 -> [w369 w394]
                  tunnel: [w368 w395] -> w359
                  tunnel: [w367 w394] -> w358
                  tunnel: w354 -> [w366 w397]
                  tunnel: [w365 w396] -> w353
                  tunnel: w349 -> [w364 w398]
                  tunnel: w348 -> [w362 _]
                  tunnel: w347 -> [w363 _]
                  frame False {
                    # "Convert to string to display"
                    n133 = for {
                      N: w362 -> [_]
                      tunnel: w370 -> [w390]
                      tunnel: [w376] -> w368
                      tunnel: w364 -> [w385]
                      shift-right: [w377] -> w367
                      shift-left: w369 -> [w389]
                      shift-right: [w386] -> w365
                      shift-left: w366 -> [w387]
                      tunnel: w363 -> [w371]
                      i -> [w380]
                      stop <- w381 stop-if-true
                      n134 = call "Send Command.vi"("error in (no error)"=w389, "Data cluster in"=w385, "VISA Refnum in"=w390) -> ("error out"=w383:errorcluster, "Data cluster out"=w382:T1, "VISA Refnum out"=w384:refnum<visa-resource-name>)  [unwired: 6 in]
                      n135 = call "Wait for Response.vi"("Timeout (ms)"=w371, "error in (no error)"=w383, "Data cluster in"=w382, "VISA Refnum in"=w384) -> ("error out"=w375:errorcluster, "Pass?"=w381:bool, "output cluster"=w374:T1, "VISA Refnum out"=w376:refnum<visa-resource-name>)  [unwired: 4 in]
                      n136 = call "Verify Response.vi"("Timeout (ms)"=w371, "error in (no error)"=w375, "output cluster in"=w374, "VISA Refnum in"=w376) -> ("error out"=w372:errorcluster, "output cluster out"=w373:T1)  [unwired: 5 in, 1 out]
                      n137 = Bundle By Name(cluster=w373, "Retries Executed"=w380) -> (w378:T1)
                      n138 = call "Decode Response.vi"("error in (no error)"=w372, "output cluster in"=w378) -> ("error out"=w377:errorcluster, "output cluster out"=w379:T1)  [unwired: 6 in]
                      n139 = call "Convert Tx Rx data to display.vi"("data cluster"=w379) -> ("Array"=w388:string[])  [unwired: 10 in]
                      n140 = Build Array (concatenate)(w387, w388) -> (w386:string[][])
                      "Data" <- w386
                    }
                  }
                  frame True {
                    # "#TODO: If more than just wait is added, then might need to loop here to search, or put instruction data elsewhere such as in command opcode data (and rename it?)"
                    # "Perform instruction step"
                    n141 = Unbundle By Name(w398) -> ("Command Name"=w393:string)
                    n142 = Match Pattern(string=w393, regular expression="Wait (ms): ") -> (match substring=w391:string)  [unwired: 1 in, 3 out]
                    n143 = case shown="\"Wait (ms): \"" w391 {
                      tunnel: w398 -> [_ w409]
                      tunnel: w397 -> [w399 w405]
                      tunnel: [w399 w403] -> w396
                      frame Default {
                      }
                      frame "Wait (ms): " {
                        # "#TODO: Theres definitely a better way to do this lol"
                        n144 = Unbundle By Name(w409) -> ("Command Name"=w408:string)
                        n145 = Search and Replace String(input string=w408, search string="Wait (ms): " ("substring (\"\")")) -> (result string=w406:string)  [unwired: 6 in, 3 out]
                        n146 = Decimal String To Number(string=w406) -> (number=w400:i32)  [unwired: 2 in, 1 out]
                        n147 = while {
                          tunnel: w400 -> [w413]
                          tunnel: w409 -> [w411]
                          tunnel: [w411] -> w402
                          stop <- w412 stop-if-true
                          n148 = Wait (ms)(milliseconds to wait=w413) -> (millisecond timer value=w410:u32)
                          n149 = Greater Or Equal?(x=w410, y=w413) -> (x >= y?=w412:bool)
                        }
                        n150 = Bundle By Name(cluster=w402, "Time (ms)"=w400) -> (w401:T1)
                        n151 = call "Convert Tx Rx data to display.vi"("data cluster"=w401) -> ("Array"=w404:string[])  [unwired: 10 in]
                        n152 = Build Array (concatenate)(w405, w404) -> (w403:string[][])
                        n153 = property on="Data" class="Tbl (strict)"("Value"=w403) -> ()  [unwired: 2 in, 2 out]
                      }
                    }
                  }
                }
              }
            }
            n154 = Enqueue Element(queue=w324, element=Main_Events."Save Data File", error in (no error)=w325) -> (queue out=w327:refnum<queue>, error out=w326:errorcluster)  [unwired: 1 in, 1 out]
          }
          frame "Save Data File" {
            # "This writes the data file at the end of the test. Could update this to write after each step or loop."
            n155 = property on="Data file path" class="Path"() -> ("Value"=w419:path)  [unwired: 2 in, 2 out]
            n156 = property on="Data" class="Tbl (strict)"() -> ("Value"=w425:string[][])  [unwired: 2 in, 2 out]
            n157 = call-poly <vilib>:"Write Delimited Spreadsheet.vi"("file path (dialog if empty)"=w419, "format (%s)"="%s", "2D data"=w425, "error in (no error)"=w422, "delimiter (\\t)"="," ("delimiter (\\t)")) -> ("error out"=w415:errorcluster)  [unwired: 9 in, 1 out]
            n158 = Path To String(path=w419) -> (string=w418:string)
            n159 = Concatenate Strings("Data saved: " ("Status"), w418) -> (w416:string)
            n160 = property on="Status" class="Str"(error in=w415, "Value"=w416) -> (error out=w414:errorcluster)  [unwired: 1 in, 1 out]
          }
        }
      }
      frame Error {
      }
    }
  }
  n161 = Release Queue(queue=w6, error in (no error)=w9) -> (error out=→"error out":errorcluster)  [unwired: 1 in, 2 out]
